vi "Motor Saftey.vi"() -> (0 "Motor Saftey":T1)   [LabVIEW 2014]
uses:
  <vilib>/Rock Robotics/WPI/SafetyOutput/WPI_SafetyOutputConfigMenu.ctl
  <vilib>/Rock Robotics/Network Tables/SD Read Boolean.vi
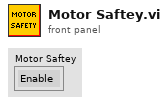
[diagram p1: front panel]
types:
  T1 = typedef "WPI_SafetyOutputConfigMenu.ctl" = enum16{"Enable", "Disable"}
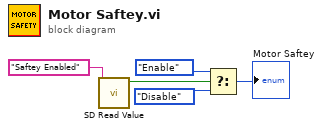
[diagram p0: block diagram]
diagram:
  n1 = call-poly <vilib>:"SD Read Value.vi"("Name"="Saftey Enabled") -> ("Boolean"=w4:bool)  [unwired: 8 in, 2 out]
  n2 = Select(t=WPI_SafetyOutputConfigMenu."Enable" ("mode"), s=w4, f=WPI_SafetyOutputConfigMenu."Disable" ("mode")) -> (s? t:f=→"Motor Saftey":T1)
